vi "WriteTDMS.vi"(9 "数据":waveform(dbl)[](array[waveform]), 10 "通道名输入（无标题）":string[](array[string])) -> ()   [LabVIEW 2013]
uses:
  GlobalValue.vi
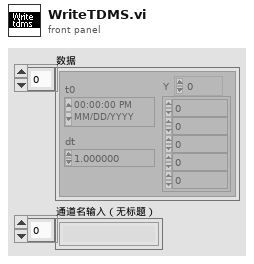
[diagram p1: front panel]
types:
  T1 = enum16{"open", "open or create", "create or replace", "create", "open (read-only)"}
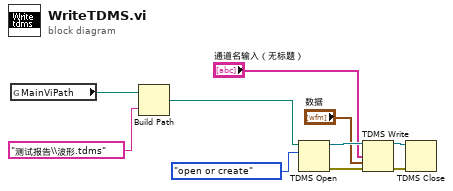
[diagram p0: block diagram]
diagram:
  n1 = global read "GlobalValue.vi" "MainViPath"() -> (w2:path)
  n2 = Build Path(base path=w2, name or relative path="测试报告\\波形.tdms" ("command line")) -> (appended path=w1:path)
  n3 = TDMS Open(10:T1."open or create" ("操作(0:open)"), 11:w1) -> (0:w9:errorcluster, 3:w6:refnum<k34>)  [unwired: 5 in]
  n4 = TDMS Write(0:w6, 7:"通道名输入（无标题）", 9:"数据", 11:w9) -> (4:w7:refnum<k34>, 15:w8:errorcluster)  [unwired: 2 in, 2 out]
  n5 = TDMS Close(8:w8, 11:w7) -> ()  [unwired: 2 out]
